vi "BIOPAC breath gating.vi"(3 "Resp Wait (ms)":u32=400) -> (1 "Resp Gate":bool caption="Silent")   [LabVIEW 2022 SP3]
doc: "I. Description:\nThis example demonstrates how to read values from one or more digital input channels.\n\nII. Instructions for Running:\n1. Select the digital lines on the DAQ device to be read.\nNote: The array indicator is sized for 8 lines, if using fewer lines, not all elements will be used. Also, if using more lines, use the array index to view elements beyond the first eight lines.\n\nIII. Block Diagram Steps:\n1. Create a Digital Input channel. Use one channel for all lines. You can alternatively use one channel for each line, but then use a different polymorphic version of the DAQmx Read VI.\n2. Call the Start VI to start the task.\n3. Read the digital data in a loop until the user hits the stop button or an error occurs. This read VI reads a single sample of digital data on demand, so no timeout is necessary.\n4. Use the Boolean Array to Number VI to view the values read as a single number\n5. Call the Clear Task VI to clear the Task.\n6. Use the popup dialog box to display an error or warning if any.\n\nIV. I/O Connections Overview:\nMake sure your signal input terminals match the Lines I/O Control. In this case wire your digital signals to the first eight digital lines on your DAQ Device."
uses:
  <vilib>/Utility/error.llb/DialogType.ctl
  <vilib>/DAQmx/read.llb/DAQmx Read (Digital Bool 1Line 1Point).vi
  <vilib>/DAQmx/create/channels.llb/DAQmx Create Channel (DI-Digital Input).vi
  <vilib>/DAQmx/miscellaneous.llb/DAQmx Fill In Error Info.vi
panel:
  in  "Lines":tag="Dev1/port2/line3"
  # "For instructions, select Help>>Show Context Help"
  # "Channel Parameters"
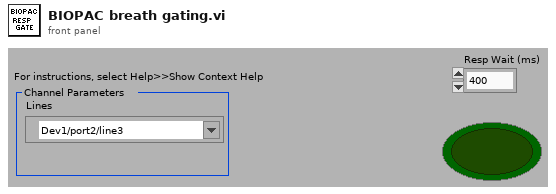
[diagram p1: front panel]
types:
  T1 = typedef "DialogType.ctl" = u16
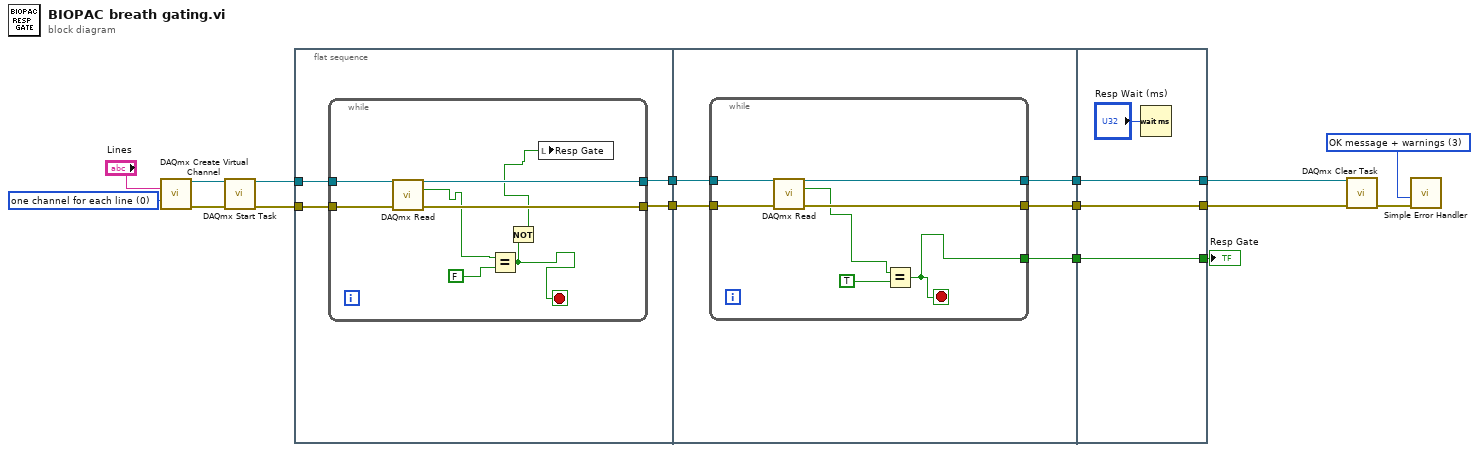
[diagram p0: block diagram]
diagram:
  w7 = 0 items=["one channel for each line", "one channel for all lines"] ("line grouping")
  w8 = T1 3 items=["no dialog", "OK message", "continue or stop message", "OK message + warnings", "continue/stop + warnings"] ("type of dialog (OK msg:1)")
  n1 = call-poly <vilib>:"DAQmx Create Virtual Channel.vi"("lines"="Lines", "line grouping"=w7) -> ("task out"=w11:refnum<k21>, "error out"=w10:errorcluster)  [unwired: 3 in, 9 out]
  n2 = call <vilib>:"DAQmx Start Task.vi"("task/channels in"=w11, "error in"=w10) -> ("task out"=w13:refnum<k21>, "error out"=w16:errorcluster)  [unwired: 12 out]
  n3 = flat-sequence {
    tunnel: w16 -> [w20]
    tunnel: w13 -> [w18]
    tunnel: [w19] -> w6
    tunnel: [w17] -> w5
    tunnel: w6 -> [w32]
    tunnel: w5 -> [w33]
    tunnel: [w30] -> w3
    tunnel: [w31] -> w2
    tunnel: [w29] -> w1
    tunnel: [w42] -> w4
    tunnel: [w43] -> w12
    tunnel: [w44] -> w15
    tunnel: w3 -> [w44]
    tunnel: w2 -> [w43]
    tunnel: w1 -> [w42]
    frame #0 {
      n4 = while {
        tunnel: w20 -> [w28]
        tunnel: [w27] -> w19
        tunnel: w18 -> [w26]
        tunnel: [w25] -> w17
        stop <- w22 stop-if-true
        n5 = call-poly <vilib>:"DAQmx Read.vi"("task/channels in"=w26, "error in"=w28) -> ("task out"=w25:refnum<k21>, "data"=w23:bool, "error out"=w27:errorcluster)  [unwired: 11 out]
        n6 = Equal?(x=w23, y=FALSE) -> (x = y?=w22:bool)
        n7 = Not(x=w22) -> (.not. x?=w21:bool)
        n8 = local write "Resp Gate"(w21) -> ()
      }
    }
    frame #1 {
      n9 = while {
        tunnel: w32 -> [w40]
        tunnel: [w39] -> w30
        tunnel: w33 -> [w38]
        tunnel: [w37] -> w31
        tunnel: [w34] -> w29
        stop <- w34 stop-if-true
        n10 = call-poly <vilib>:"DAQmx Read.vi"("task/channels in"=w38, "error in"=w40) -> ("task out"=w37:refnum<k21>, "data"=w35:bool, "error out"=w39:errorcluster)  [unwired: 11 out]
        n11 = Equal?(x=w35, y=TRUE) -> (x = y?=w34:bool)
      }
    }
    frame #2 {
      n12 = Wait (ms)(milliseconds to wait="Resp Wait (ms)") -> ()  [unwired: 1 out]
    }
  }
  n13 = call <vilib>:"DAQmx Clear Task.vi"("task in"=w12, "error in"=w15) -> ("error out"=w14:errorcluster)  [unwired: 13 out]
  n14 = call <vilib>:"Simple Error Handler.vi"("type of dialog (OK msg:1)"=w8, "error in (no error)"=w14) -> ()  [unwired: 8 out]
  "Resp Gate" <- w4
